vi "Commit Properties.vi"(0 "Session Handle in":T1, 5 "resources":string, 11 "error in (no error)":errorcluster) -> (4 "Session Handle out":T1, 15 "error out":errorcluster)   [LabVIEW 2015, in "SLSC Switch.lvlib" / "SLSC Session.lvclass"]
uses:
  SLSC Session.lvclass
  Typedefs/Session Handle.ctl
  SLSC Session.lvclass/SLSC Session.ctl
  <vilib>/SLSC/SLSC.lvlib
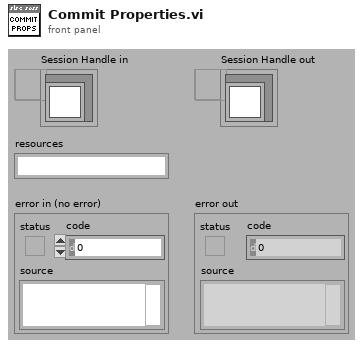
[diagram p1: front panel]
types:
  T1 = typedef "SLSC Switch.lvlib/SLSC Session.lvclass/Session Handle.ctl" = refnum<data-value>
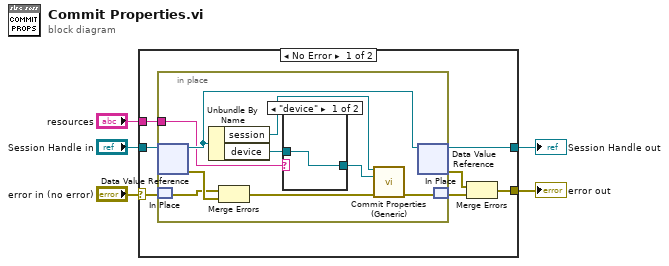
[diagram p0: block diagram]
diagram:
  n1 = case shown="No Error" "error in (no error)" {
    selector: "error in (no error)" -> [w7 w24]
    tunnel: "Session Handle in" -> [w12 w25]
    tunnel: [w11 w25] -> w4
    tunnel: [w8 w24] -> w3
    tunnel: "resources" -> [w6 _]
    frame No Error {
      n2 = in-place {
        in-place-border: w6 -> [w15]
        n3 = in-place-dvr #1(w12) -> (w19:refnum<class "SLSC Session.lvclass">, w21:errorcluster)
        n4 = in-place-match #2(w7) -> (w20:errorcluster)
        n5 = Unbundle By Name(w19) -> ("session"=w18:refnum<k21>, "device"=w13:refnum<k21>)
        n6 = Merge Errors(w20, w21) -> (w17:errorcluster)
        n7 = case shown="\"device\"" w15 {
          selector: w15 -> [_ w23]
          tunnel: [w22 w23] -> w14
          tunnel: w13 -> [w22 _]
          frame "device" {
          }
          frame Default {
          }
        }
        n8 = call <vilib>:"Commit Properties (Generic).vi"("session in"=w18, "resources"=w14, "error in (no error)"=w17) -> ("error out"=w16:errorcluster)  [unwired: 11 in, 1 out]
        n9 = in-place-dvr #1(w19) -> (w11:T1, w9:errorcluster)
        n10 = in-place-match #2(w16) -> (w10:errorcluster)
      }
      n11 = Merge Errors(w9, w10) -> (w8:errorcluster)
    }
    frame Error {
    }
  }
  "Session Handle out" <- w4
  "error out" <- w3
